vi "Teleop.vi"(10 "Match Info":T1={"Autonomous Elapsed Seconds"=0.0, "TeleOp Elapsed Seconds"=0.0, "Disabled Elapsed Seconds"=0.0, "Visited Autonomous"=FALSE, "Visited TeleOp"=FALSE, "Visited Disabled"=FALSE, "Autonomous Settings"={"Autonomous Style"=enum."Independent", "VI Refnum"=refnum}}, 11 "Call Context":T2) -> ()   [LabVIEW 2015]
doc: "This VI is called for each enabled TeleOp packet received from the DS. It is typically used to read from joysticks and other inputs and update I/O or setpoints for timed control loops. It should complete and return within 20 milliseconds or risk missing DS packets."
uses:
  <vilib>/Rock Robotics/WPI/DriverStation/WPI_DriverStationDerivedRobotMode.ctl
  <vilib>/Rock Robotics/WPI/DriverStation/WPI_DriverStationMatch Info.ctl
  Handling/Implementation/Handling Operations.ctl
  Support Code/Logitech/F510/F510-X.vi
  Handling/Implementation/Handling Published Globals.vi
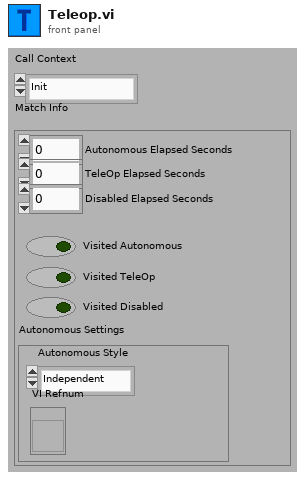
[diagram p1: front panel]
types:
  T1 = typedef "WPI_DriverStationMatch Info.ctl" = cluster{"Autonomous Elapsed Seconds":dbl, "TeleOp Elapsed Seconds":dbl, "Disabled Elapsed Seconds":dbl, "Visited Autonomous":bool, "Visited TeleOp":bool, "Visited Disabled":bool, "Autonomous Settings":cluster{"Autonomous Style":enum16{"Iterative", "Independent"}, "VI Refnum":refnum<vi>}}
  T2 = typedef "WPI_DriverStationDerivedRobotMode.ctl" = enum16{"Init", "Execute", "Stop"}
  T3 = cluster{"A":bool, "B":bool, "X":bool, "Y":bool, "LB":bool, "RB":bool, "Back":bool, "Start":bool, "LC":bool, "RC":bool, "LT":bool, "RT":bool}
  T4 = cluster{"Up":bool, "Right":bool, "Down":bool, "Left":bool}
  T5 = typedef "Handling Operations.ctl" = enum16{"Reserve", "Read Current", "Pickup Ball", "Fire"}
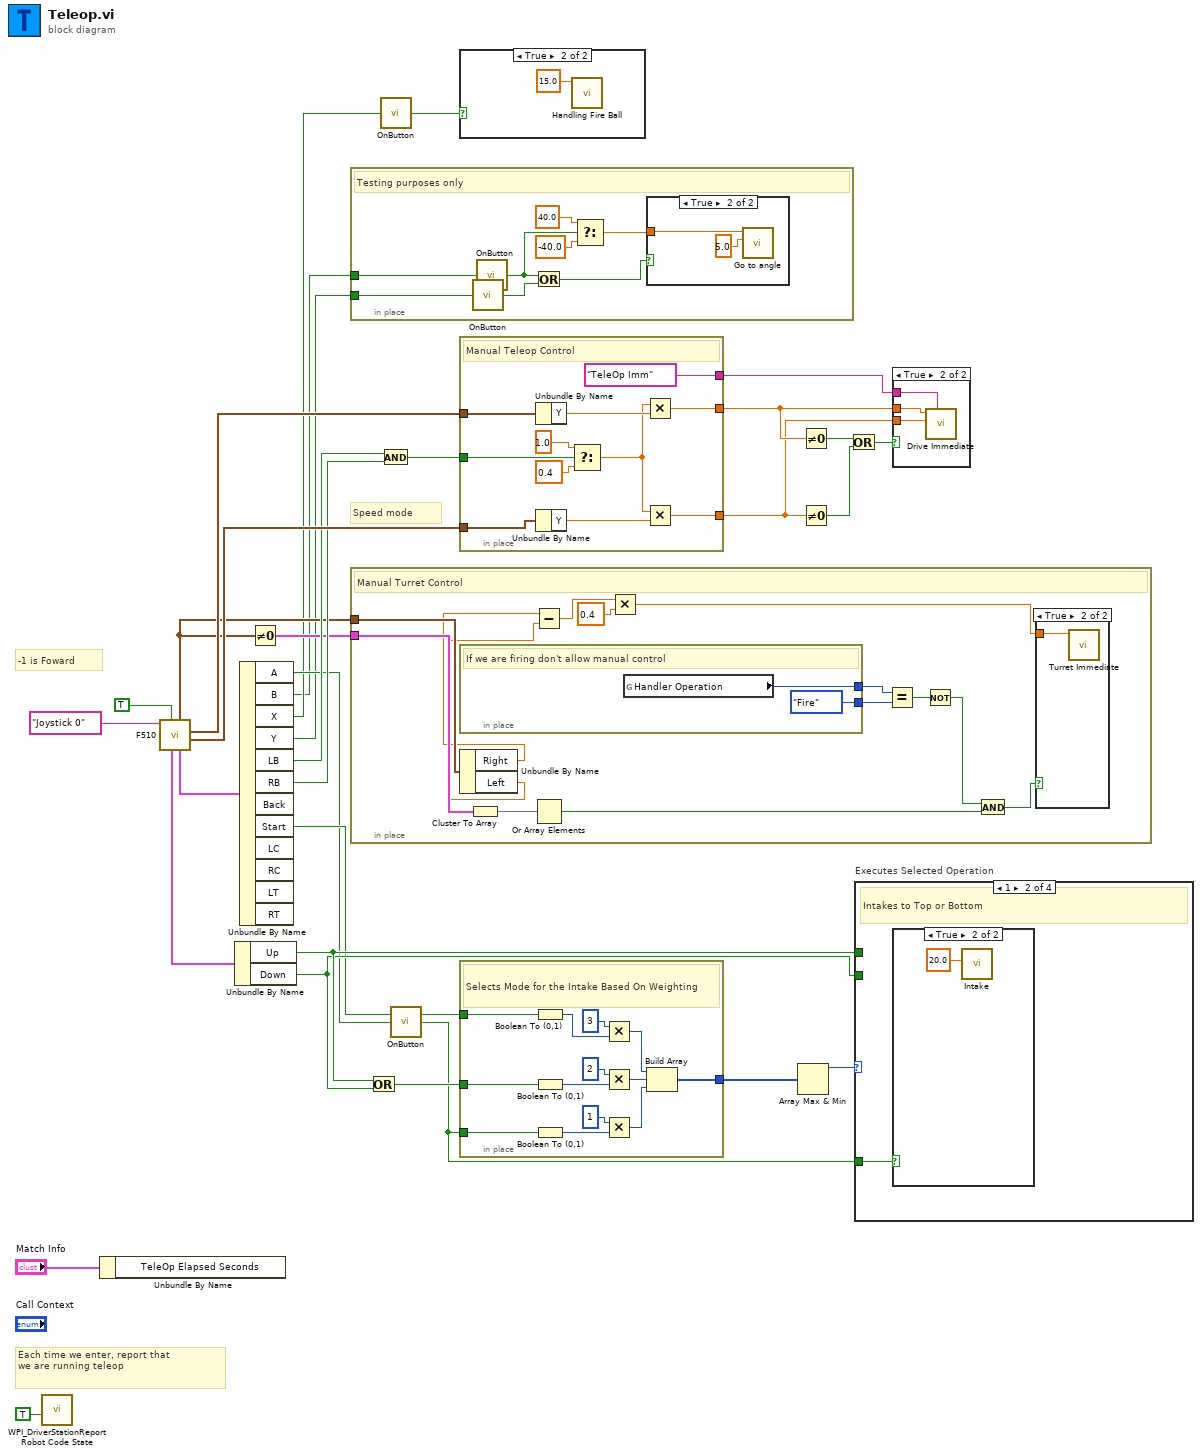
[diagram p0: block diagram]
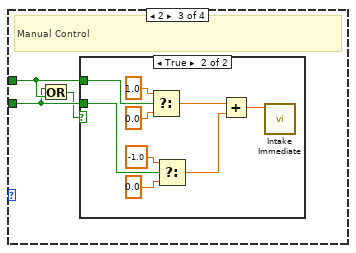
[diagram p8: hidden frame]
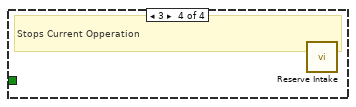
[diagram p10: hidden frame]
diagram:
  # "-1 is Foward"
  # "Speed mode"
  # "Each time we enter, report that\nwe are running teleop"
  n1 = call <vilib>:"WPI_DriverStationReport Robot Code State.vi"("TeleOp"=TRUE ("Autonomous")) -> ()  [unwired: 10 in, 1 out]
  n2 = Unbundle By Name("Match Info") -> ()  [unwired: 1 out]
  n3 = call-poly "F510.vi"("Smooth Control (T)"=TRUE, "refnum name"="Joystick 0") -> ("Right Stick"=w27:cluster{"X":dbl, "Y":dbl}, "Left Stick"=w28:cluster{"X":dbl, "Y":dbl}, "Buttons"=w25:T3, "Triggers"=w10:cluster{"Left":dbl, "Right":dbl}, "D-Pad Buttons"=w21:T4)  [unwired: 3 in, 2 out]
  n4 = Unbundle By Name(w21) -> ("Up"=w20:bool, "Down"=w19:bool)
  n5 = Unbundle By Name(w25) -> ("A"=w16:bool, "B"=w6:bool, "X"=w8:bool, "Y"=w7:bool, "LB"=w23:bool, "RB"=w24:bool, "Start"=w17:bool)  [unwired: 5 out]
  n6 = Not Equal To 0?(x=w10) -> (x != 0?=w11:cluster{"Left":bool, "Right":bool})
  n7 = in-place {
    in-place-border: w6 -> [w34]
    in-place-border: w7 -> [w33]
    # "Testing purposes only"
    n8 = call "OnButton.vi"("Button"=w33) -> ("Value"=w32:bool)  [unwired: 1 in]
    n9 = call "OnButton.vi"("Button"=w34) -> ("Value"=w35:bool)  [unwired: 1 in]
    n10 = Or(x=w35, y=w32) -> (x .or. y?=w36:bool)
    n11 = Select(t=40.0 ("x"), s=w35, f=-40.0 ("x")) -> (s? t:f=w38:dbl)
    n12 = case shown="True" w36 {
      tunnel: w38 -> [_ w41]
      frame False {
      }
      frame True {
        n13 = call "Go to angle.vi"("Duration"=5.0, "Angle  (degrees, 0=straight ahead)"=w41) -> ()  [unwired: 9 in, 1 out]
      }
    }
  }
  n14 = in-place {
    in-place-border: w11 -> [w55]
    in-place-border: w10 -> [w45]
    # "Manual Turret Control"
    n15 = in-place {
      in-place-border: [w56] -> w50
      in-place-border: [Handling_Operations."Fire" ("y")] -> w49
      # "If we are firing don't allow manual control"
      n16 = global read "Handling Published Globals.vi" "Handler Operation"() -> (w56:T5)
    }
    n17 = Unbundle By Name(w45) -> ("Right"=w43:dbl, "Left"=w42:dbl)
    n18 = Cluster To Array(cluster=w55) -> (array=w53:bool[])
    n19 = Subtract(x=w43, y=w42) -> (x-y=w44:dbl)
    n20 = Or Array Elements(Boolean array=w53) -> (logical OR=w54:bool)
    n21 = Multiply(x=w44, y=0.4) -> (x*y=w46:dbl)
    n22 = Equal?(x=w50, y=w49) -> (x = y?=w48:bool)
    n23 = Not(x=w48) -> (.not. x?=w51:bool)
    n24 = And(x=w51, y=w54) -> (x .and. y?=w52:bool)
    n25 = case shown="True" w52 {
      tunnel: w46 -> [_ w58]
      frame False {
      }
      frame True {
        n26 = call "Turret Immediate.vi"("Speed (-1 to 1)"=w58) -> ()  [unwired: 10 in, 1 out]
      }
    }
  }
  n27 = Or(x=w20, y=w19) -> (x .or. y?=w18:bool)
  n28 = call "OnButton.vi"("Button"=w8) -> ("Value"=w9:bool)  [unwired: 1 in]
  n29 = And(x=w23, y=w24) -> (x .and. y?=w22:bool)
  n30 = call "OnButton.vi"("Button"=w16) -> ("Value"=w13:bool)  [unwired: 1 in]
  n31 = case shown="True" w9 {
    frame False {
    }
    frame True {
      n32 = call "Handling Fire Ball.vi"("Duration"=15.0) -> ()  [unwired: 10 in, 1 out]
    }
  }
  n33 = in-place {
    in-place-border: w28 -> [w70]
    in-place-border: w27 -> [w69]
    in-place-border: w22 -> [w66]
    in-place-border: ["TeleOp Imm" ("Description")] -> w12
    in-place-border: [w61] -> w3
    in-place-border: [w60] -> w2
    # "Manual Teleop Control"
    n34 = Unbundle By Name(w70) -> ("Y"=w68:dbl)
    n35 = Unbundle By Name(w69) -> ("Y"=w67:dbl)
    n36 = Select(t=1.0, s=w66, f=0.4) -> (s? t:f=w63:dbl)
    n37 = Multiply(x=w63, y=w68) -> (x*y=w61:dbl)
    n38 = Multiply(x=w63, y=w67) -> (x*y=w60:dbl)
  }
  n39 = in-place {
    in-place-border: w18 -> [w82]
    in-place-border: w17 -> [w77]
    in-place-border: [w72] -> w15
    in-place-border: w13 -> [w71]
    # "Selects Mode for the Intake Based On Weighting"
    n40 = Boolean To (0,1)(Boolean=w77) -> (0, 1=w79:i16)
    n41 = Boolean To (0,1)(Boolean=w82) -> (0, 1=w83:i16)
    n42 = Boolean To (0,1)(Boolean=w71) -> (0, 1=w75:i16)
    n43 = Multiply(x=i16 3, y=w79) -> (x*y=w76:i16)
    n44 = Multiply(x=i16 2, y=w83) -> (x*y=w80:i16)
    n45 = Multiply(x=i16 1, y=w75) -> (x*y=w73:i16)
    n46 = Build Array(w76, w80, w73) -> (w72:i16[])
  }
  n47 = Array Max & Min(array=w15) -> (max value=w14:i16)  [unwired: 3 out]
  n48 = Not Equal To 0?(x=w3) -> (x != 0?=w4:bool)
  n49 = Not Equal To 0?(x=w2) -> (x != 0?=w1:bool)
  n50 = Or(x=w4, y=w1) -> (x .or. y?=w5:bool)
  n51 = case "Executes Selected Operation" shown="1" w14 {
    tunnel: w20 -> [_ _ w88 _]
    tunnel: w19 -> [_ _ w87 _]
    tunnel: w13 -> [_ w84 _ _]
    frame 0, Default {
      # "Nothing"
    }
    frame 1 {
      # "Intakes to Top or Bottom"
      n52 = case shown="True" w84 {
        frame False {
        }
        frame True {
          n53 = call "Intake.vi"("Duration (s)"=20.0) -> ()  [unwired: 10 in, 1 out]
        }
      }
    }
    frame 2 {
      # "Manual Control"
      n54 = Or(x=w87, y=w88) -> (x .or. y?=w86:bool)
      n55 = case shown="True" w86 {
        tunnel: w88 -> [_ w97]
        tunnel: w87 -> [_ w96]
        frame False {
        }
        frame True {
          n56 = Select(t=1.0, s=w97, f=0.0) -> (s? t:f=w90:dbl)
          n57 = Select(t=-1.0, s=w96, f=0.0) -> (s? t:f=w91:dbl)
          n58 = Add(x=w90, y=w91) -> (x+y=w89:dbl)
          n59 = call "Intake Immediate.vi"("Setpoint"=w89) -> ()  [unwired: 10 in, 1 out]
        }
      }
    }
    frame 3 {
      # "Stops Current Opperation"
      n60 = call "Reserve Intake.vi"() -> ()  [unwired: 11 in, 1 out]
    }
  }
  n61 = case shown="True" w5 {
    tunnel: w12 -> [_ w100]
    tunnel: w2 -> [_ w99]
    tunnel: w3 -> [_ w98]
    frame False {
    }
    frame True {
      n62 = call "Drive Immediate.vi"("Description"=w100, "Right Setpoint"=w99, "Left Setpoint"=w98) -> ()  [unwired: 8 in, 1 out]
    }
  }
